vi "Check and Execute Burst Cell.vi"(0 "1D Board":T1[](array[typedef]), 11 "error in (no error)":errorcluster) -> (4 "1D Board Out":T1[](array[typedef]), 15 "error out":errorcluster)   [LabVIEW 2014, in "Dragon Tamers.lvlib"]
uses:
  Typedefs/Board Cell.ctl
  Typedefs/Cell Occupancy.ctl
  Dragon Tamers.lvlib
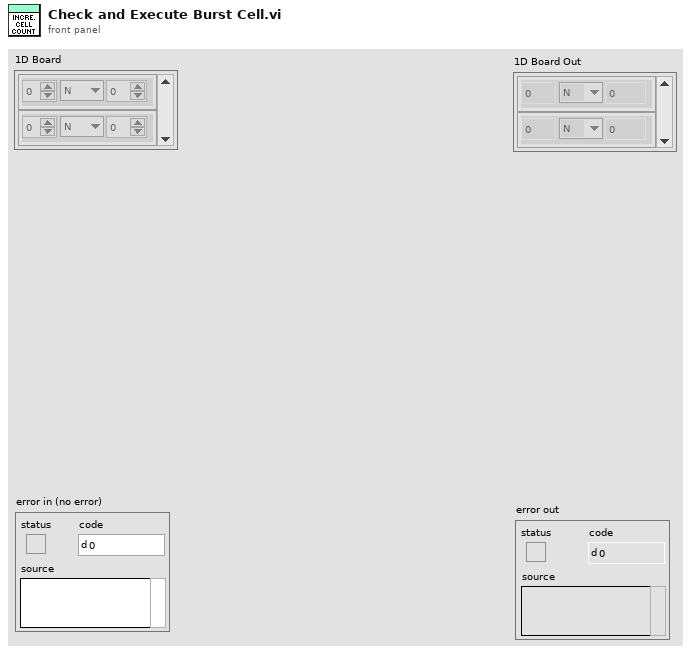
[diagram p1: front panel]
types:
  T1 = typedef "Dragon Tamers.lvlib/Board Cell.ctl" = cluster{"Team":i32, "Occu.":T2, "Count":i32}
  T2 = typedef "Dragon Tamers.lvlib/Cell Occupancy.ctl" = enum16{"N", "C", "K"}
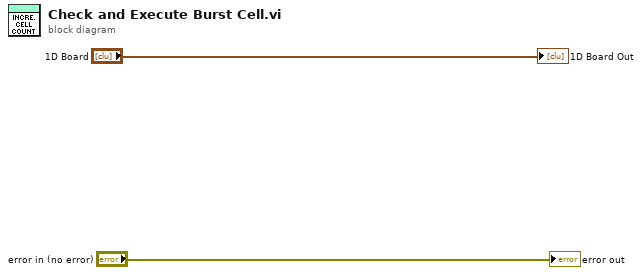
[diagram p0: block diagram]
diagram:
  "error out" <- "error in (no error)"
  "1D Board Out" <- "1D Board"
